vi "Get Process ID From FPGA.vi"(8 "error in (no error)":errorcluster, 10 "FPGA Name":string, 11 "Tamer in":refnum<class "Tamer.lvclass">) -> (0 "error out":errorcluster, 2 "Process ID":string, 3 "Tamer out":refnum<class "Tamer.lvclass">)   [LabVIEW 2020, in "Tamer.lvlib" / "Tamer.lvclass"]
uses:
  Tamer.lvclass
  TALOS/TALOS_PPL.lvlibp
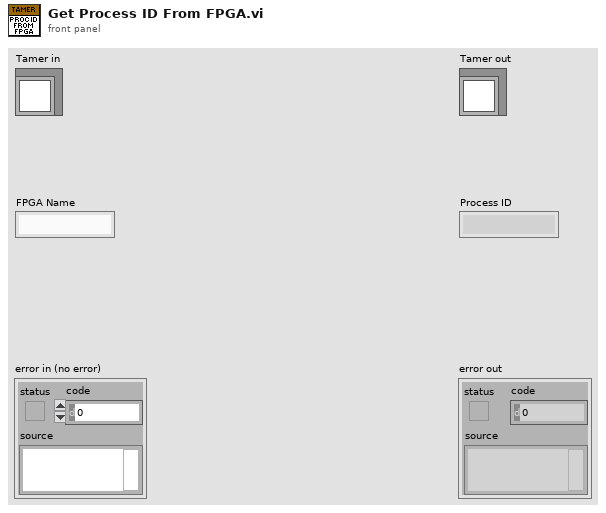
[diagram p1: front panel]
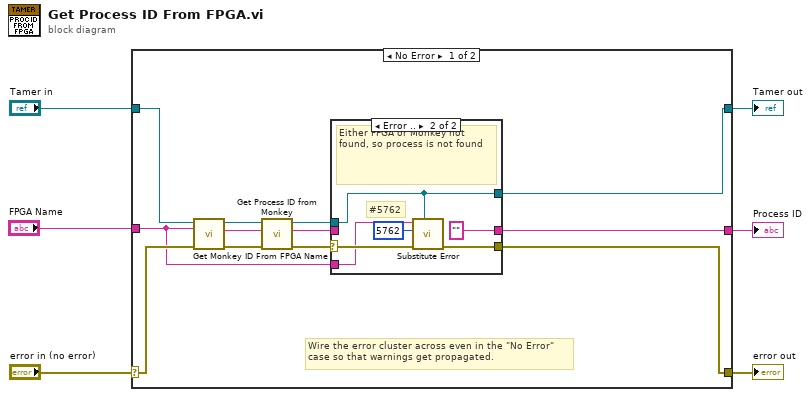
[diagram p0: block diagram]
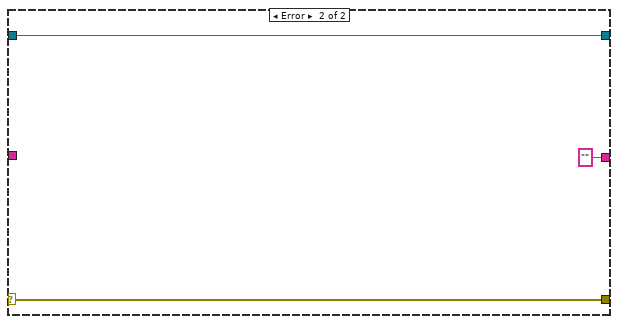
[diagram p3: hidden frame]
diagram:
  n1 = case shown="No Error" "error in (no error)" {
    selector: "error in (no error)" -> [w16 w30]
    tunnel: [w8 w30] -> w5
    tunnel: [w9 w29] -> w3
    tunnel: "Tamer in" -> [w18 w29]
    tunnel: "FPGA Name" -> [w10 _]
    tunnel: [w7 "" ("Process ID")] -> w1
    frame No Error {
      # "Wire the error cluster across even in the \"No Error\"\ncase so that warnings get propagated."
      n2 = call-dynamic "Get Monkey ID From FPGA Name.vi"("error in (no error)"=w16, "FPGA Name"=w10, "Tamer in"=w18) -> ("error out"=w15:errorcluster, "Monkey ID"=w17:string, "Tamer out"=w14:refnum<class "Tamer.lvclass">)  [unwired: 6 in]
      n3 = call-dynamic "Get Process ID from Monkey.vi"("error in (no error)"=w15, "Monkey ID"=w17, "Tamer in"=w14) -> ("error out"=w13:errorcluster, "Process ID"=w11:string, "Tamer out"=w12:refnum<class "Tamer.lvclass">)  [unwired: 6 in]
      n4 = case shown="Error .." w13 {
        selector: w13 -> [w20 w27]
        tunnel: w12 -> [w21 w24]
        tunnel: w11 -> [w19 _]
        tunnel: w10 -> [_ w26]
        tunnel: [w21 w24] -> w9
        tunnel: [w20 w23] -> w8
        tunnel: [w19 "" ("Process ID")] -> w7
        frame No Error {
          # "All good"
        }
        frame Error {
          # "#5762"
          # "Either FPGA or Monkey not found, so process is not found"
          n5 = call "Substitute Error.vi"("LabVIEW Object"=w24, "error in (no error)"=w27, "Error Code"=5762, "Optional String"=w26) -> ("error out"=w23:errorcluster)  [unwired: 7 in]
        }
      }
    }
    frame Error {
    }
  }
  "error out" <- w5
  "Tamer out" <- w3
  "Process ID" <- w1
